vi "DigGageData.vi"(0 "Machine Params":T7 {"Scan Info"."sector scan angle" format="%.2f"; "Scan Info"."pivot distance" format="%.2f"; "Scan Info"."delay" format="%.2f"}, 1 "Counter Params":T9={"Cal (F)/Acq (T) Counters"=FALSE, "Macine Type"=enum."B&K Hawk"}, 3 "Vecchio Hitachi?":bool, 5 "Digitizer Settings":T1={"Digitizer delay (us) "=0.0, "rf points per line"=2048, "lines per plane"=128, "Samp Rate (Hz)"=100000000.0, "Additional dig delay (us)"=0.0, "Voltage Scale"=0.4, "Pre-Looks"=0, "Offset delay (us)"=0.0, "bits A/D"=8, "Avg Num"=1, "DigTimeOut"=5.0, "Rel Dig Delay"=0.0, "Dig Ch"=0, "LeCroyCluster"={"LeCroy Channels"=[TRUE, FALSE, FALSE, FALSE], "LC read pt offset"=0.0, "Sweep Avg"=FALSE}, "Main Digitizer"=enum."NI Digitizer", "Dig Config"=enum."Single channel", "Digitizer ID Cluster"={"Acqiris/Alazar/SP ID"=[], "NI Instr Handles"=[], "LeCroy VISA"="", "GaGe Handle"={"Handle"=0, "Sample size"=0, "Resolution"=0, "Offset"=0, "Channels"=0, "Boards"=0}, "ATS Ref"="ATS9350", "Acqiris Address"=["PCI::INSTR0"], "ADQRef"=refnum, "adq_cu_ptr"=refnum}, "Trigger Settings"={"Trig Source"=1, "Trig Coupling"=0, "Trig Slope"=0, "Level (mV)"=1500.0}, "Bulk Acq"=FALSE, "Bulk Start Indexes"=[], "Data Ref RF"=refnum, "NI ID/Channel"=[], "Total Dig CH"=5, "Xtra Ann Trig delay (us)"=10.0, "Fix Z Delay?"=FALSE, "One Way Transmission?"=FALSE, "Data Ref Log"=refnum} {"Trigger Settings"."Trig Slope" items=["Positive", "Negative"]; "Trigger Settings"."Level (mV)" format="%.2f"; "Trigger Settings"."Trig Coupling" items=["DC 1 MOhm", "AC 1 MOhm", "DC 50 Ohm", "AC 50 Ohm"]; "Trigger Settings"."Trig Source" items=["Chan 1", "External"]; "Rel Dig Delay" format="%.2f"; "DigTimeOut" format="%.2f"; "Avg Num" min=1; "Offset delay (us)" format="%.2f"; "Additional dig delay (us)" format="%.2f"; "Digitizer delay (us)" format="%.2f"}, 9 "Frame Prams":cluster{"Divide By":u8, "frames":i32}, 11 "Patient Info":T8={"ID"="", "Extended ID"="", "age"=0, "gender"="", "previously\nscanned"="N", "PSA"=0.0, "LOS"=1, "Ethnicty"=3, "Race"=3} {"Race" items=["Am Ind or Alaska", "Asian", "Hawaiian, Pac Isl", "Black or Afr Amer", "White", "more than one race", "unknown"]; "Ethnicty" items=["Hispanic", "Non-Hispanic", "unknown"]; "LOS" items=["1", "2", "3", "4", "5"]; "PSA" format="%.1f"}, 12 "File Name":string, 14 "Attenuation":u8(slide) max=63 scale=0.0..63.0) -> (4 "output cluster":T6={"header info"={"Header"="", "Head length"=0}, "A/D info"={"# rf points per line"=0, "# lines per scan"=0, "sample rate MHz"=0, "# A/D bits"=0, "# bytes per A/D"=0, "TGC Flag"=0, "A/D Type"=""}, "Tranducer Info"={"bandwidth"=0.0, "center freq"=0.0, "start freq"=0.0, "ID"=0}, "Scan Info"={"delay"=0.0, "pivot distance"=0.0, "sector scan angle"=0.0, "operator"="", "Scan Mode"="", "location"=""}, "Time/Date Info"={"date"="", "time"=""}, "RF Info"={"RF file name"="", "RF file att"="", "RF cal file name"="", "RF cal file att"=""}, "Patient Info"={"ID"="", "extended ID"="", "age"=0, "sex"="", "previously\nscanned"="", "PSA"=0.0, "LOS"=1, "Ethnicty 2"=3, "Race"=3}, "Tissue Type"={"organ"=0, "disease type"=0, "disease location"=0, "IQ_pts"=0, "RcvBuffer"=0, "RcvFrame"=0, "IQBuff"=0, "IQFrame"=0, "IQPage"=0}, "Votage scaling"={"Digitizer (dB)"=0.0, "Gain (dB)"=0.0, "Atten (dB)"=0.0}, "Comment"="", "Misc Info"={"avg num"=0, "c speed"=0, "Div By or SF zones"=0, "XMIT CHS"=0, "RCV CHS"=0, "Xmit angle"=0.0}, "Therapy Parameters"={"Theraputic Freq (MHz)"=0.1, "Time on (s)"=1.0, "Therapy amplitude (mV)"=50.0, "Lines Before"=20, "Lines After"=80}, "Scan Settings"={"Energy (uJ or V)"=0, "Damp (Ohm) or Fc"=0, "HP Filt (KHz)"=0, "LP Filt (MHz)"=0, "Gain (db)"=0, "prf (kHz)"=0.0, "Distance between\nscan lines (um)"=0, "Distance between\nscan planes (um)"=0, "Scan line gap (um)"=0.0, "Scan plane gap (um)"=0.0}, "Compression Parameters"={"F1 (MHz)"=0.0, "F2 (MHz)"=0.0, "% taper"=0.0, "duration"=0.0}, "Patient Info Xtra"={"First Name"="", "Last Name"="", "Notes"=""}, "ROI Box"=[0, 0, 0, 0]} {"Compression Parameters"."% taper" min=50 max=1000 format="%.2f"; "Compression Parameters"."F2 (MHz)" format="%.3f"; "Compression Parameters"."F1 (MHz)" format="%.3f"; "Scan Settings"."prf (kHz)" format="%.2f"; "Therapy Parameters"."Therapy amplitude (mV)" min=50 max=1000 format="%.2f"; "Therapy Parameters"."Time on (s)" format="%.3f"; "Therapy Parameters"."Theraputic Freq (MHz)" format="%.3f"; "Patient Info"."Race" items=["Am Ind or Alaska", "Asian", "Hawaiian, Pac Isl", "Black or Afr Amer", "White", "more than one race", "unknown"]; "Patient Info"."Ethnicty 2" items=["Hispanic", "Non-Hispanic", "unknown"]; "Patient Info"."LOS" items=["1", "2", "3", "4", "5"]; "Patient Info"."PSA" format="%.1f"; "Scan Info"."delay" format="%.2f"; "Scan Info"."pivot distance" format="%.2f"; "Scan Info"."sector scan angle" format="%.2f"; "Tranducer Info"."bandwidth" format="%.2f"; "Tranducer Info"."center freq" format="%.2f"; "Tranducer Info"."start freq" format="%.2f"}, 6 "Data":i16[][][](array[numeric]), 8 "Scan Params":T5, 10 "TGC data":i16[][](array[numeric]), 13 "Array":picture[](array[picture]), 15 "Error Message":string)   [LabVIEW 2022 SP3]
uses:
  <instrlib>/vi.lib/Platform/portaccess.llb/Out Port8.vi
  ViewData/-ReadEye/Header.ctl
  MachineParams.ctl
  ScanningControl/Digitizers/-DigitizerRoutines/DigitizerID.ctl
  ScanningControl/Digitizers/-DigitizerRoutines/DigitizerSettings.ctl
  ScanningControl/Digitizers/-DigitizerRoutines/Digitizer.ctl
  ScanningControl/Digitizers/-DigitizerRoutines/DigConfig.ctl
  C:/Windows/System32/ADQAPI_dotNet_helper.dll
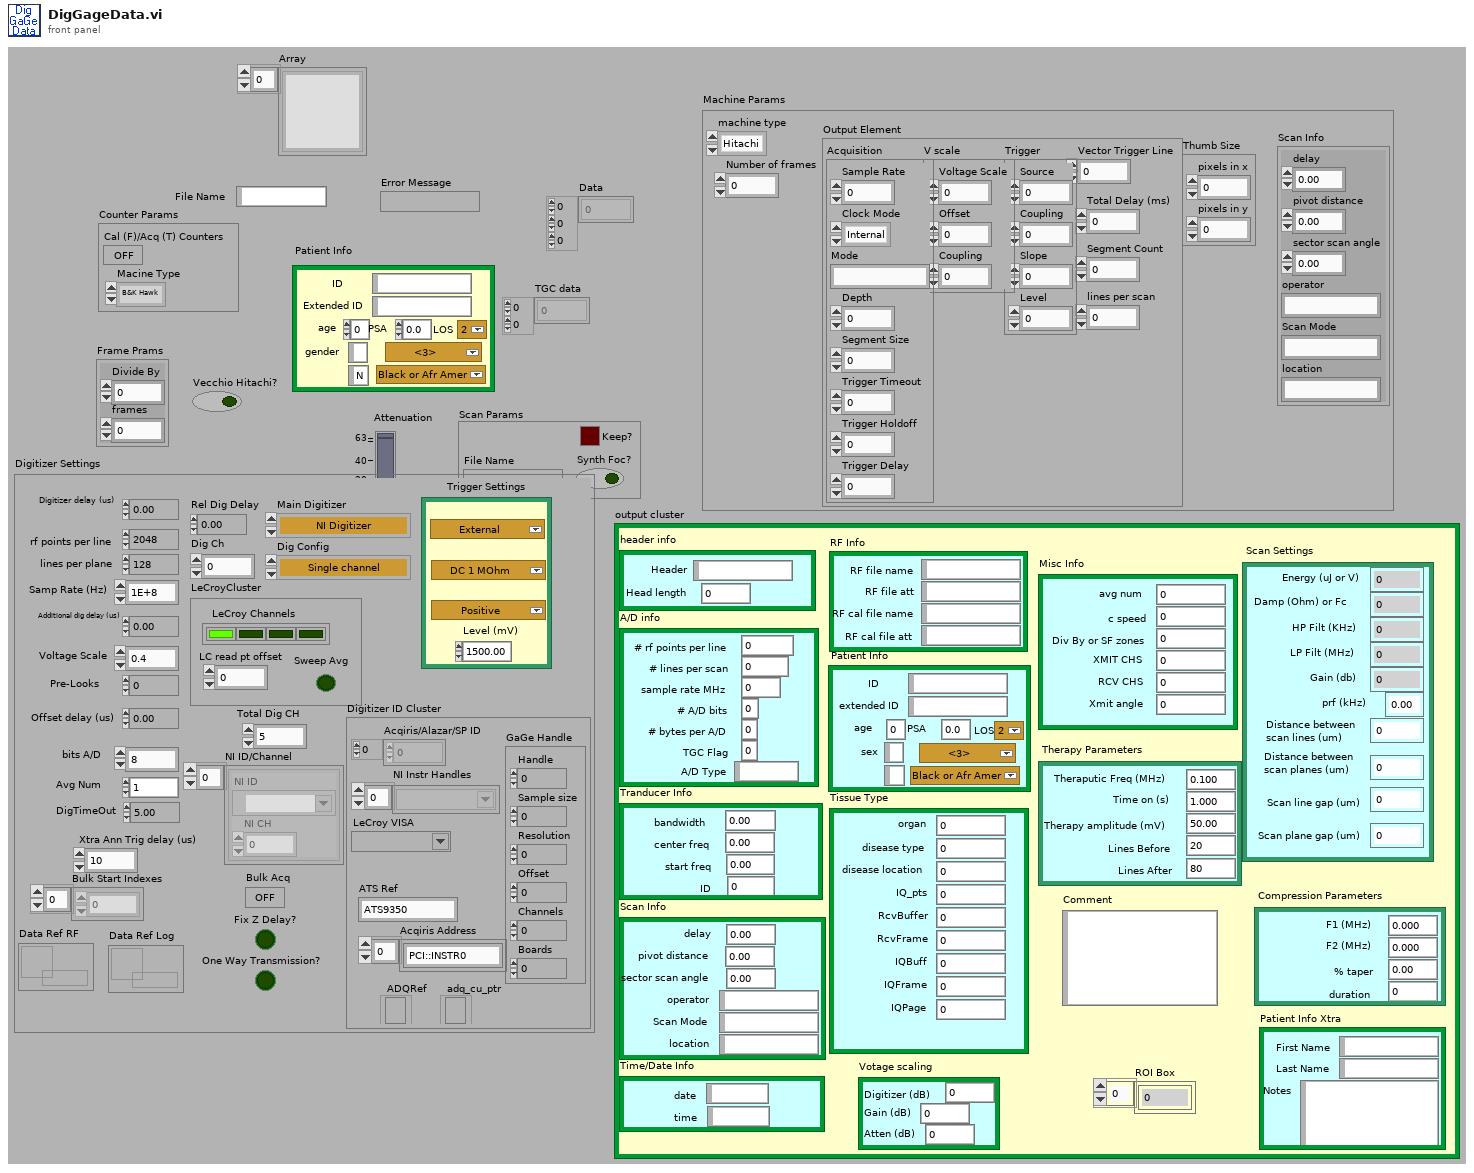
[diagram p1: front panel]
types:
  T1 = typedef "DigitizerSettings.ctl" = cluster{"Digitizer delay (us) ":dbl, "rf points per line":i32, "lines per plane":i32, "Samp Rate (Hz)":dbl, "Additional dig delay (us)":dbl, "Voltage Scale":dbl, "Pre-Looks":i32, "Offset delay (us)":dbl, "bits A/D":i8, "Avg Num":i32, "DigTimeOut":sgl, "Rel Dig Delay":sgl, "Dig Ch":i32, "LeCroyCluster":cluster{"LeCroy Channels":bool[], "LC read pt offset":dbl, "Sweep Avg":bool}, "Main Digitizer":T2, "Dig Config":T3, "Digitizer ID Cluster":T4, "Trigger Settings":cluster{"Trig Source":u16, "Trig Coupling":u16, "Trig Slope":u16, "Level (mV)":dbl}, "Bulk Acq":bool, "Bulk Start Indexes":i32[], "Data Ref RF":refnum<data-value>, "NI ID/Channel":cluster{"NI ID":refnum<k15>, "NI CH":i32}[], "Total Dig CH":i32, "Xtra Ann Trig delay (us)":dbl, "Fix Z Delay?":bool, "One Way Transmission?":bool, "Data Ref Log":refnum<data-value>}
  T2 = typedef "Digitizer.ctl" = enum16{"Acqiris Digitizer", "NI Digitizer", "LeCroy", "GaGe", "AlazarTech", "No Digitizer", "Teledyne"}
  T3 = typedef "DigConfig.ctl" = enum16{"Single channel", "2 Chans w/ 2 Acqiris", "2 Chans w/ 1 Acqiris", "5-CH Pulser New", "5-CH pulser w/ ann array", "5-pass style ann array", "Empty"}
  T4 = typedef "DigitizerID.ctl" = cluster{"Acqiris/Alazar/SP ID":u32[], "NI Instr Handles":refnum<k15>[], "LeCroy VISA":refnum<visa-resource-name>, "GaGe Handle":cluster{"Handle":u32, "Sample size":u32, "Resolution":i32, "Offset":i32, "Channels":u32, "Boards":u32}, "ATS Ref":string, "Acqiris Address":string[], "ADQRef":refnum<k24>, "adq_cu_ptr":refnum<k24>}
  T5 = cluster{"File Name":string, "Keep?":bool, "Synth Foc?":bool}
  T6 = typedef "Header.ctl" = cluster{"header info":cluster{"Header":string, "Head length":i16}, "A/D info":cluster{"# rf points per line":u16, "# lines per scan":u16, "sample rate MHz":u16, "# A/D bits":i16, "# bytes per A/D":u16, "TGC Flag":u16, "A/D Type":string}, "Tranducer Info":cluster{"bandwidth":sgl, "center freq":sgl, "start freq":sgl, "ID":i32}, "Scan Info":cluster{"delay":sgl, "pivot distance":sgl, "sector scan angle":sgl, "operator":string, "Scan Mode":string, "location":string}, "Time/Date Info":cluster{"date":string, "time":string}, "RF Info":cluster{"RF file name":string, "RF file att":string, "RF cal file name":string, "RF cal file att":string}, "Patient Info":cluster{"ID":string, "extended ID":string, "age":u16, "sex":string, "previously\nscanned":string, "PSA":sgl, "LOS":u8, "Ethnicty 2":u8, "Race":u8}, "Tissue Type":cluster{"organ":i16, "disease type":i16, "disease location":i16, "IQ_pts":u16, "RcvBuffer":u8, "RcvFrame":u16, "IQBuff":u8, "IQFrame":u16, "IQPage":u8}, "Votage scaling":cluster{"Digitizer (dB)":sgl, "Gain (dB)":sgl, "Atten (dB)":sgl}, "Comment":string, "Misc Info":cluster{"avg num":u16, "c speed":i16, "Div By or SF zones":i16, "XMIT CHS":u8, "RCV CHS":u8, "Xmit angle":sgl}, "Therapy Parameters":cluster{"Theraputic Freq (MHz)":sgl, "Time on (s)":sgl, "Therapy amplitude (mV)":sgl, "Lines Before":u16, "Lines After":u16}, "Scan Settings":cluster{"Energy (uJ or V)":u8, "Damp (Ohm) or Fc":u8, "HP Filt (KHz)":u8, "LP Filt (MHz)":u8, "Gain (db)":u8, "prf (kHz)":sgl, "Distance between\nscan lines (um)":u16, "Distance between\nscan planes (um)":u16, "Scan line gap (um)":sgl, "Scan plane gap (um)":sgl}, "Compression Parameters":cluster{"F1 (MHz)":sgl, "F2 (MHz)":sgl, "% taper":sgl, "duration":sgl}, "Patient Info Xtra":cluster{"First Name":string, "Last Name":string, "Notes":string}, "ROI Box":u16[]}
  T7 = typedef "MachineParams.ctl" = cluster{"machine type":enum16{"Hitachi", "B&K 3535", "B&K Hawk"}, "Number of frames":dbl, "Output Element":cluster{"Acquisition":cluster{"Sample Rate":dbl, "Clock Mode":enum16{"Internal", "External", "Reference"}, "Mode":string, "Depth":dbl, "Segment Size":dbl, "Trigger Timeout":dbl, "Trigger Holdoff":dbl, "Trigger Delay":dbl}, "V scale":cluster{"Voltage Scale":i16, "Offset":dbl, "Coupling":u16}, "Trigger":cluster{"Source":u16, "Coupling":u16, "Slope":u16, "Level":dbl}, "Vector Trigger Line":i16, "Total Delay (ms)":dbl, "Segment Count":u32, "lines per scan":i32}, "Thumb Size":cluster{"pixels in x":i16, "pixels in y":i16}, "Scan Info":cluster{"delay":sgl, "pivot distance":sgl, "sector scan angle":sgl, "operator":string, "Scan Mode":string, "location":string}}
  T8 = cluster{"ID":string, "Extended ID":string, "age":u16, "gender":string, "previously\nscanned":string, "PSA":sgl, "LOS":u8, "Ethnicty":u8, "Race":u8}
  T9 = cluster{"Cal (F)/Acq (T) Counters":bool, "Macine Type":enum16{"Hitachi", "B&K 3535", "B&K Hawk"}}
  T10 = cluster{"Handle":u32, "Sample size":u32, "Resolution":i32, "Offset":i32, "Channels":u32, "Boards":u32}
  T11 = cluster{"Voltage Scale":i16, "Offset":dbl, "Coupling":u16}
  T12 = cluster{"Source":u16, "Coupling":u16, "Slope":u16, "Level":dbl}
  T13 = cluster{"Sample Rate":dbl, "Clock Mode":enum16{"Internal", "External", "Reference"}, "Mode":string, "Depth":dbl, "Segment Size":dbl, "Trigger Timeout":dbl, "Trigger Holdoff":dbl, "Trigger Delay":dbl}
  T14 = cluster{sgl, "Gain [dB]  ":sgl, "Atten (dB)":sgl}
  T15 = typedef "Header.ctl" = cluster{"header info":cluster{"Header":string, "Head length":i16}, "A/D info":cluster{"# rf points per line":u16, "# lines per scan":u16, "sample rate MHz":u16, "# A/D bits":i16, "# bytes per A/D":u16, "TGC Flag":u16, "A/D Type":string}, "Tranducer Info":cluster{"bandwidth":sgl, "center freq":sgl, "start freq":sgl, "ID":i32}, "Scan Info":cluster{"delay":sgl, "pivot distance":sgl, "sector scan angle":sgl, "operator":string, "Scan Mode":string, "location":string}, "Time/Date Info":cluster{"date":string, "time":string}, "RF Info":cluster{"RF file name":string, "RF file att":string, "RF cal file name":string, "RF cal file att":string}, "Patient Info":cluster{"ID":string, "extended ID":string, "age":u16, "sex":string, "previously\nscanned":string, "PSA":sgl, "LOS":u8, "Ethnicty 2":u8, "Race":u8}, "Tissue Type":cluster{"organ":i16, "disease type":i16, "disease location":i16, "IQ_pts":u16, "RcvBuffer":u8, "RcvFrame":u16, "IQBuff":u8, "IQFrame":u16, "IQPage":u8}, "Votage scaling":cluster{"Digitizer (dB)":sgl, "Gain (dB)":sgl, "Atten (dB)":sgl}, "Comment":string, "Misc Info":cluster{"avg num":u16, "c speed":i16, "Div By or SF zones":i16, "XMIT CHS":u8, "RCV CHS":u8, "Xmit angle":sgl}, "Therapy Parameters":cluster{"Theraputic Freq (MHz)":sgl, "Time on (s)":sgl, "Therapy amplitude (mV)":sgl, "Lines Before":u16, "Lines After":u16}, "Scan Settings":cluster{"Energy (uJ or V)":u8, "Damp (Ohm) or Fc":u8, "HP Filt (KHz)":u8, "LP Filt (MHz)":u8, "Gain (db)":u8, "prf (kHz)":sgl, "Distance between\nscan lines (um)":u16, "Distance between\nscan planes (um)":u16}, "Compression Parameters":cluster{"F1 (MHz)":sgl, "F2 (MHz)":sgl, "% taper":sgl, "duration":sgl}, "Patient Info Xtra":cluster{"First Name":string, "Last Name":string, "Notes":string}, "ROI Box":u16[]}
  T16 = cluster{"delay":sgl, "pivot distance":sgl, "sector scan angle":sgl, "operator":string, "Scan Mode":string, "location":string}
  T17 = cluster{"File Name":string, "Synth Foc?":bool, "Synth Foc?":bool}
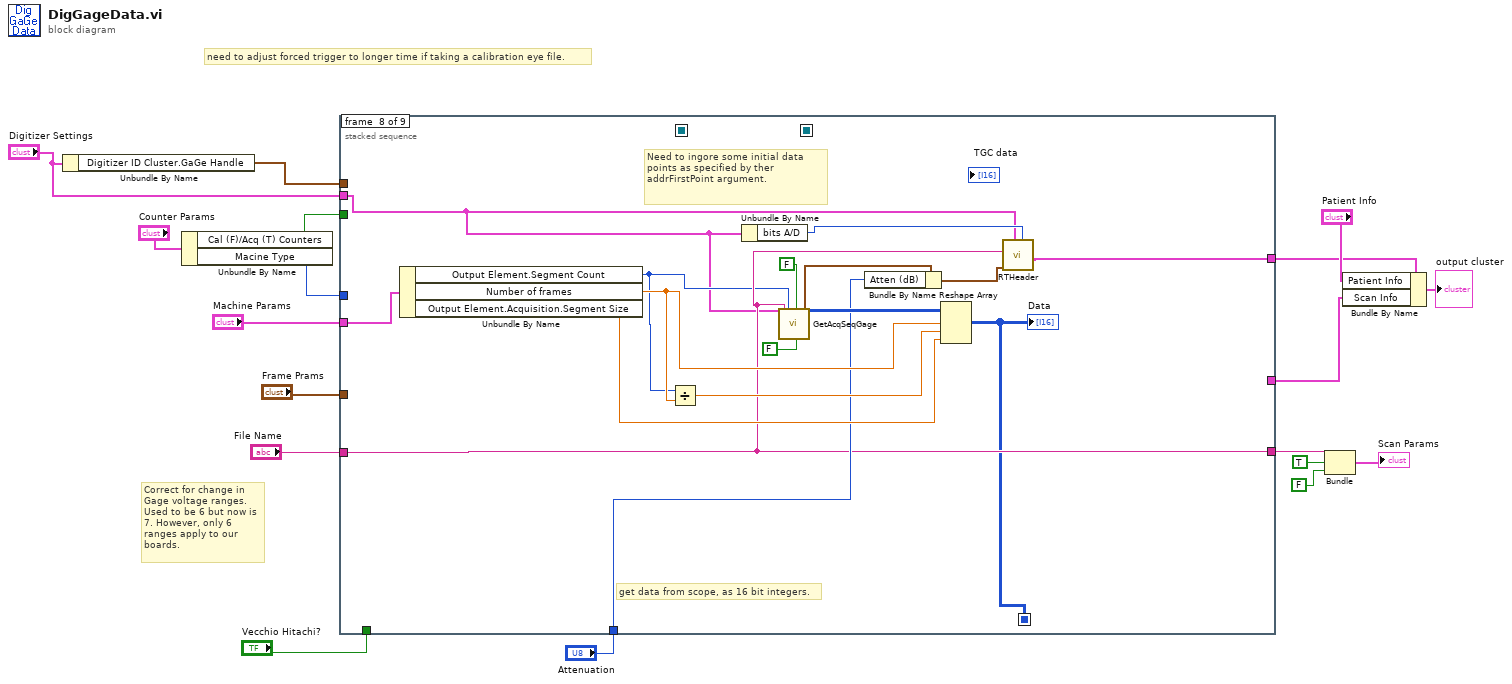
[diagram p0: block diagram]
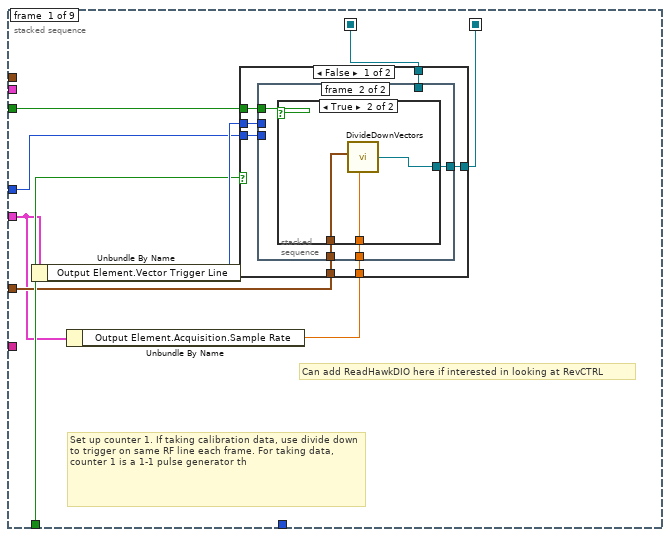
[diagram p2: hidden frame]
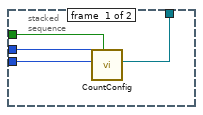
[diagram p3: hidden frame]
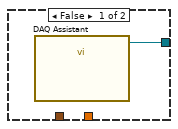
[diagram p4: hidden frame]
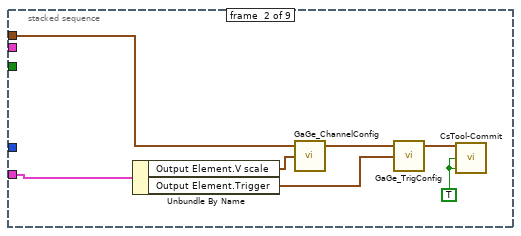
[diagram p6: hidden frame]
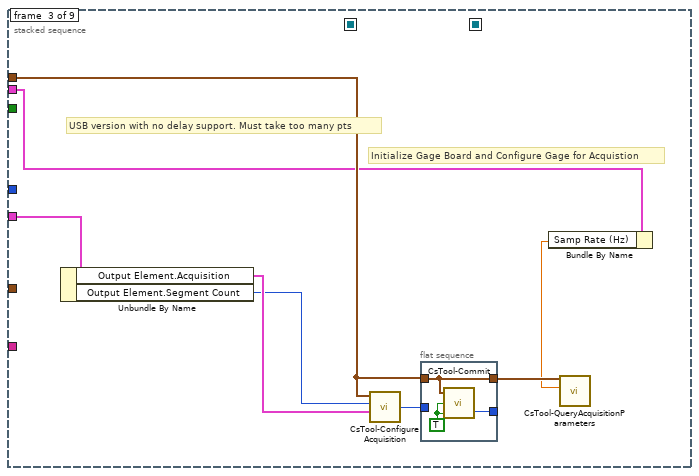
[diagram p7: hidden frame]
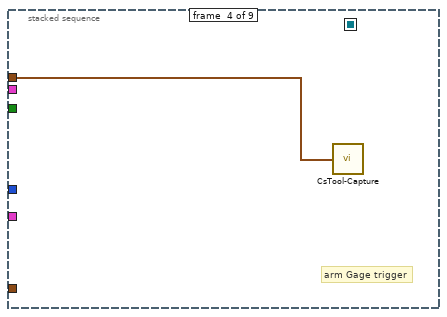
[diagram p8: hidden frame]
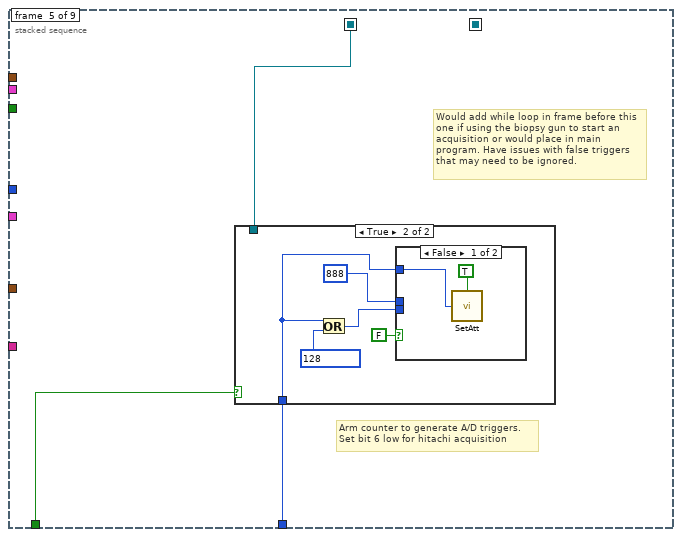
[diagram p9: hidden frame]
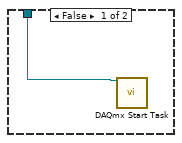
[diagram p10: hidden frame]
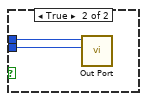
[diagram p11: hidden frame]
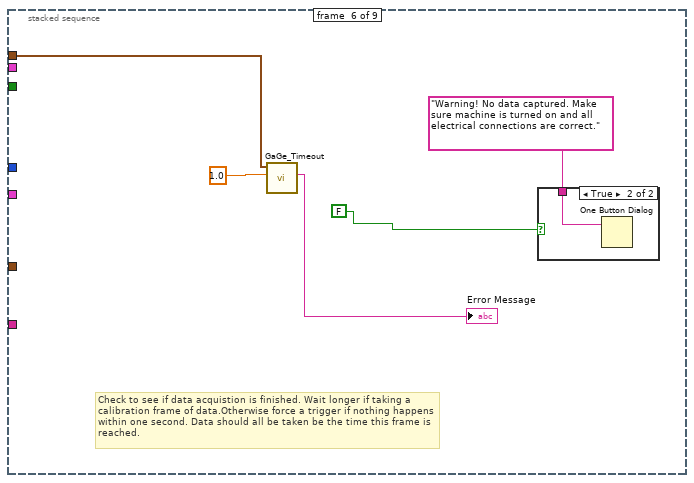
[diagram p12: hidden frame]
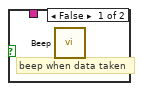
[diagram p13: hidden frame]
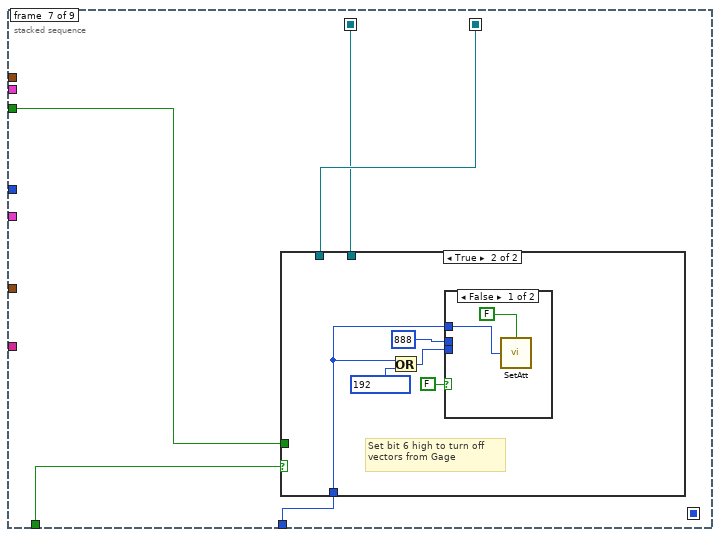
[diagram p14: hidden frame]
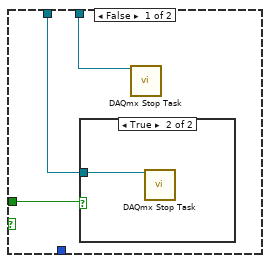
[diagram p15: hidden frame]
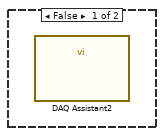
[diagram p16: hidden frame]
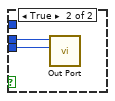
[diagram p17: hidden frame]
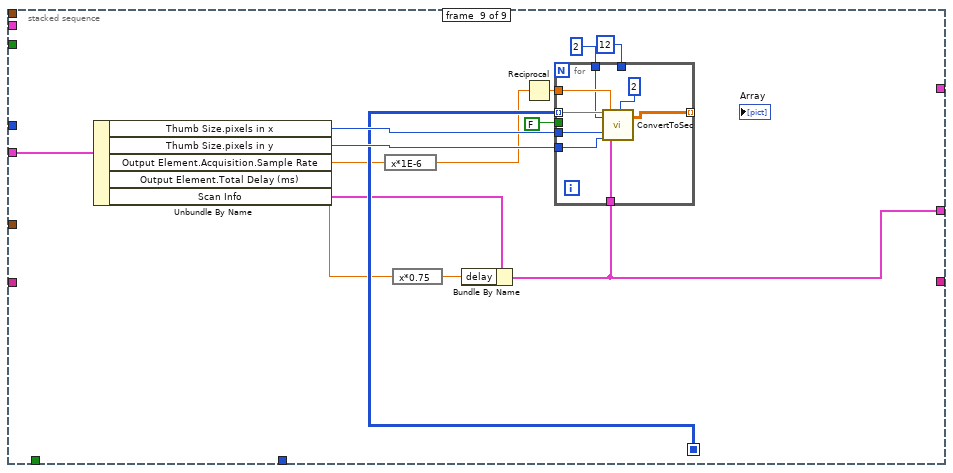
[diagram p18: hidden frame]
diagram:
  # "Correct for change in Gage voltage ranges. Used to be 6 but now is 7. However, only 6 ranges apply to our boards."
  # "need to adjust forced trigger to longer time if taking a calibration eye file."
  n1 = Unbundle By Name("Digitizer Settings") -> ("Digitizer ID Cluster.GaGe Handle"=w2:T10)
  n2 = Unbundle By Name("Counter Params") -> ("Cal (F)/Acq (T) Counters"=w17:bool, "Macine Type"=w16:enum16{"Hitachi", "B&K 3535", "B&K Hawk"})
  n3 = stacked-sequence {
    seq-local: [w21 _ _ _ _ _ _ _ _] -> [_ _ _ _ _ _ w86 _ _]
    seq-local: [w20 _ _ _ _ _ _ _ _] -> [_ _ _ _ w66 _ w85 _ _]
    seq-local: [_ _ _ _ _ _ _ w106 _] -> [_ _ _ _ _ _ _ _ w129]
    tunnel: "Machine Params" -> [w19 w49 w59 _ _ _ _ w107 w132]
    tunnel: w17 -> [w27 _ _ _ _ _ w87 _ _]
    tunnel: w16 -> [w25 _ _ _ _ _ _ _ _]
    tunnel: "Vecchio Hitachi?" -> [w24 _ _ _ w68 _ w89 _ _]
    tunnel: "Attenuation" -> [_ _ _ _ w67 _ w88 w110 _]
    tunnel: "Frame Prams" -> [w23 _ _ _ _ _ _ _ _]
    tunnel: w2 -> [_ w50 w60 w65 _ w81 _ _ _]
    tunnel: "File Name" -> [_ _ _ _ _ _ _ w109 _]
    tunnel: [_ _ _ _ _ _ _ w109 _] -> w10
    tunnel: [_ _ _ _ _ _ _ w105 _] -> w4
    tunnel: [_ _ _ _ _ _ _ _ w119] -> w3
    tunnel: "Digitizer Settings" -> [_ _ w55 _ _ _ _ w103 _]
    frame #0 {
      # "Can add ReadHawkDIO here if interested in looking at RevCTRL"
      # "Set up counter 1. If taking calibration data, use divide down to trigger on same RF line each frame. For taking data, counter 1 is a 1-1 pulse generator th"
      n4 = Unbundle By Name(w19) -> ("Output Element.Vector Trigger Line"=w26:i16)
      n5 = Unbundle By Name(w19) -> ("Output Element.Acquisition.Sample Rate"=w22:dbl)
      n6 = case shown="False" w24 {
        tunnel: w27 -> [w34 _]
        tunnel: w26 -> [w33 _]
        tunnel: w25 -> [w32 _]
        tunnel: w23 -> [w31 _]
        tunnel: w22 -> [w30 _]
        tunnel: [w29 _] -> w21
        tunnel: [w28 _] -> w20
        frame False {
          n7 = stacked-sequence {
            tunnel: w34 -> [w38 w40]
            tunnel: w33 -> [w37 _]
            tunnel: w32 -> [w36 _]
            tunnel: w31 -> [_ w42]
            tunnel: w30 -> [_ w41]
            tunnel: [_ w39] -> w29
            tunnel: [w35 _] -> w28
            frame #0 {
              n8 = call "CountConfig.vi"("Cal (F)/Acq (T) Counters"=w38, "Machine Type"=w36, "pulse delay  (cycles)"=w37) -> ("task out"=w35:refnum<k21>)  [unwired: 8 out]
            }
            frame #1 {
              n9 = case shown="True" w40 {
                tunnel: w42 -> [_ w46]
                tunnel: w41 -> [_ w45]
                tunnel: [w43 w44] -> w39
                frame False {
                  n10 = call "DAQ Assistant"() -> ("task out"=w43:refnum<k21>)  [unwired: 3 in, 16 out]
                }
                frame True {
                  n11 = call "DivideDownVectors.vi"("Frame Prams"=w46, "Total Lines"=w45) -> ("task out"=w44:refnum<k21>)  [unwired: 5 out]
                }
              }
            }
          }
        }
        frame True {
        }
      }
    }
    frame #1 {
      w52 = TRUE
      n12 = Unbundle By Name(w49) -> ("Output Element.V scale"=w47:T11, "Output Element.Trigger"=w48:T12)
      n13 = call "GaGe_ChannelConfig.vi"("V scale"=w47, "Handle Cluster"=w50) -> ("Handle Cluster Out"=w53:T10)  [unwired: 3 in]
      n14 = call "GaGe_TrigConfig.vi"("Trigger"=w48, "Handle Cluster"=w53) -> ("Handle Cluster Out"=w51:T10)  [unwired: 3 in]
      n15 = call <userlib>:"CsTool-Commit.vi"("OnlyOnChange (t)"=w52, "Coerce Flag (f)"=w52, "Handle Cluster"=w51) -> ()  [unwired: 2 out]
    }
    frame #2 {
      # "USB version with no delay support. Must take too many pts"
      # "Initialize Gage Board and Configure Gage for Acquistion"
      n16 = Unbundle By Name(w59) -> ("Output Element.Acquisition"=w58:T13, "Output Element.Segment Count"=w57:u32)
      n17 = call <userlib>:"CsTool-ConfigureAcquisition.vi"("Handle Cluster"=w60, "Segment Count (1)"=w57, "Acquisition"=w58) -> ("Error Code"=w61:i32)  [unwired: 2 in]
      n18 = flat-sequence {
        tunnel: [w62] -> w56
        tunnel: w60 -> [w62]
        tunnel: [w63] -> _
        tunnel: w61 -> [_]
        frame #0 {
          w64 = TRUE
          n19 = call <userlib>:"CsTool-Commit.vi"("OnlyOnChange (t)"=w64, "Coerce Flag (f)"=w64, "Handle Cluster"=w62) -> ("Error Code"=w63:i32)  [unwired: 1 out]
        }
      }
      n20 = call <userlib>:"CsTool-QueryAcquisitionParameters.vi"("Handle Cluster"=w56) -> ("Sample Rate"=w54:dbl)  [unwired: 10 out]
      n21 = Bundle By Name(cluster=w55, "Samp Rate (Hz)"=w54) -> ()  [unwired: 1 out]
    }
    frame #3 {
      # "arm Gage trigger"
      n22 = call <userlib>:"CsTool-Capture.vi"("Handle Cluster"=w65) -> ()  [unwired: 1 out]
    }
    frame #4 {
      # "Would add while loop in frame before this one if using the biopsy gun to start an acquisition or would place in main program. Have issues with false triggers that may need to be ignored."
      # "Arm counter to generate A/D triggers.\nSet bit 6 low for hitachi acquisition"
      n23 = case shown="True" w68 {
        tunnel: w67 -> [_ w70]
        tunnel: w66 -> [w69 _]
        frame False {
          n24 = call <vilib>:"DAQmx Start Task.vi"("task/channels in"=w69) -> ()  [unwired: 1 in, 14 out]
        }
        frame True {
          n25 = Or(x=w70, y=u8 128) -> (x .or. y?=w74:u8)
          n26 = case shown="False" FALSE {
            tunnel: w74 -> [_ w78]
            tunnel: u32 888 ("Port Address") -> [_ w77]
            tunnel: w70 -> [w75 _]
            frame False {
              n27 = call "SetAtt.vi"("Arm Trigs?"=TRUE, "Attenuation"=w75) -> ()  [unwired: 4 in]
            }
            frame True {
              n28 = call-poly <instrlib>:"Out Port.vi"("write value"=w78, "address"=w77) -> ()  [unwired: 1 in, 7 out]
            }
          }
        }
      }
    }
    frame #5 {
      # "Check to see if data acquistion is finished. Wait longer if taking a calibration frame of data.Otherwise force a trigger if nothing happens within one second. Data should all be taken be the time this frame is reached."
      n29 = call "GaGe_Timeout.vi"("TimeOut (s)"=sgl 1.0, "GaGe Handle"=w81) -> ("String"=→"Error Message":string)  [unwired: 8 in, 1 out]
      n30 = case shown="True" FALSE {
        tunnel: "Warning! No data captured. Make sure machine is turned on and all electrical connections are correct." -> [_ w84]
        frame False {
          # "beep when data taken"
          n31 = call <vilib>:"Beep.vi"() -> ()  [unwired: 3 in, 9 out]
        }
        frame True {
          n32 = One Button Dialog(message=w84) -> ()  [unwired: 2 out]
        }
      }
    }
    frame #6 {
      n33 = case shown="True" w89 {
        tunnel: w88 -> [_ w94]
        tunnel: w87 -> [w92 _]
        tunnel: w86 -> [w91 _]
        tunnel: w85 -> [w90 _]
        frame False {
          n34 = case shown="True" w92 {
            tunnel: w91 -> [_ w93]
            frame False {
              n35 = call "DAQ Assistant2"() -> ()  [unwired: 3 in, 17 out]
            }
            frame True {
              n36 = call <vilib>:"DAQmx Stop Task.vi"("task/channels in"=w93) -> ()  [unwired: 1 in, 14 out]
            }
          }
          n37 = call <vilib>:"DAQmx Stop Task.vi"("task/channels in"=w90) -> ()  [unwired: 1 in, 14 out]
        }
        frame True {
          # "Set bit 6 high to turn off vectors from Gage"
          n38 = Or(x=w94, y=u8 192) -> (x .or. y?=w98:u8)
          n39 = case shown="False" FALSE {
            tunnel: w98 -> [_ w102]
            tunnel: u32 888 ("Port Address") -> [_ w101]
            tunnel: w94 -> [w100 _]
            frame False {
              n40 = call "SetAtt.vi"("Arm Trigs?"=FALSE, "Attenuation"=w100) -> ()  [unwired: 4 in]
            }
            frame True {
              n41 = call-poly <instrlib>:"Out Port.vi"("write value"=w102, "address"=w101) -> ()  [unwired: 1 in, 7 out]
            }
          }
        }
      }
    }
    frame #7 {
      # "get data from scope, as 16 bit integers."
      # "Need to ingore some initial data points as specified by ther addrFirstPoint argument."
      n42 = Unbundle By Name(w107) -> ("Output Element.Segment Count"=w108:u32, "Number of frames"=w115:dbl, "Output Element.Acquisition.Segment Size"=w113:dbl)
      n43 = Divide(x=w108, y=w115) -> (x/y=w114:dbl)
      n44 = Unbundle By Name(w103) -> ("bits A/D"=w104:i8)
      n45 = call "GetAcqSeqGage.vi"("Digitizer Settings"=w103, "Numbered File"=w109, "lines per plane"=w108, "save?"=FALSE, "Reverse?"=FALSE) -> ("Voltage Scale"=w112:T14, "Array"=w116:i16[][])  [unwired: 19 in, 2 out]
      n46 = Bundle By Name(cluster=w112, "Atten (dB)"=w110) -> (w111:T14)
      n47 = Reshape Array(w116, w115, w114, w113) -> (w106:i16[][][])
      "Data" <- w106
      n48 = call "RTHeader.vi"("Dig Word Size"=w104, "Digitizer Settings"=w103, "Votage scaling"=w111, "File Name In"=w109) -> ("Header Out"=w105:T15)  [unwired: 6 in, 1 out]
    }
    frame #8 {
      n49 = Unbundle By Name(w132) -> ("Thumb Size.pixels in x"=w131:i16, "Thumb Size.pixels in y"=w130:i16, "Output Element.Acquisition.Sample Rate"=w128:dbl, "Output Element.Total Delay (ms)"=w121:dbl, "Scan Info"=w122:T16)
      n50 = expression code="x*1E-6"(w128) -> (w127:dbl)
      n51 = expression code="x*0.75"(w121) -> (w120:dbl)
      n52 = Bundle By Name(cluster=w122, "delay"=w120) -> (w119:T16)
      n53 = Reciprocal(x=w127) -> (1/x=w126:dbl)
      n54 = for {
        tunnel: w131 -> [w140]
        tunnel: w130 -> [w139]
        tunnel: w129 -> [w138] mode=indexing
        tunnel: w126 -> [w137]
        tunnel: 12 -> [_]
        tunnel: FALSE ("no oversample?") -> [_]
        tunnel: 2 -> [w135]
        tunnel: w119 -> [w134]
        tunnel: [w133] -> _ mode=indexing
        n55 = call "ConvertToSec.vi"("raw image data in"=w138, "reduce pts by factor of"=w135, "pixels in x"=w140, "pixels in y"=w139, "Time between rf pts\nmicros"=w137, "Scan Info"=w134, "Smooth factor"=2) -> ("raw sector out"=w133:dbl[][])  [unwired: 4 in, 8 out]
      }
    }
  }
  n56 = Bundle("File Name"=w10, "Synth Foc?"=TRUE, "Synth Foc?"=FALSE) -> (→"Scan Params":T17)  [unwired: 1 in]
  n57 = Bundle By Name(cluster=w4, "Patient Info"="Patient Info", "Scan Info"=w3) -> (→"output cluster":T15)
